vi "Message to Message Handler.vi"(0 "Message Handler In":refnum<class "Message Handler.lvclass">, 1 "CMD":T2, 2 "Type of Message":T1, 5 "Process":refnum<class "Process.lvclass">, 7 "Data In":variant, 9 "Return State":string, 11 "Error In":errorcluster, 12 "Timeout in ms (-1)":i32) -> (4 "Message Handler Out":refnum<class "Message Handler.lvclass">, 8 "Data Out":variant, 15 "Error Out":errorcluster)   [LabVIEW 2023, in "Message Handler.lvclass"]
uses:
  Message Handler.lvclass
  Public/Ctrls/CMDs.ctl
  Process/Process.lvclass
  Public/Ctrls/Type of Message.ctl
  Process/Process.lvclass/Process.ctl
  Message Handler.lvclass/Message Handler.ctl
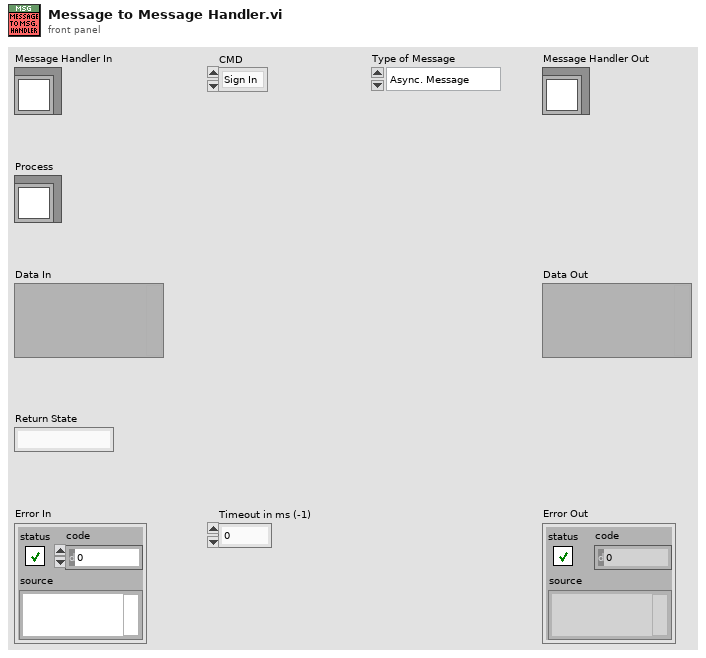
[diagram p1: front panel]
types:
  T1 = typedef "Message Handler.lvclass/Type of Message.ctl" = enum16{"Async. Message", "Async. Data Request", "Sync. Data Request"}
  T2 = typedef "Message Handler.lvclass/CMDs.ctl" = enum16{"Sign In"}
  T3 = typedef "ICanCommunicate.lvclass/Message.ctl" = cluster{"Sender Name":string, "Recipent Name":string, "Command":string, "Data":variant, "Time Stamp":timestamp, "GUID":string, "Chcecksum":string}
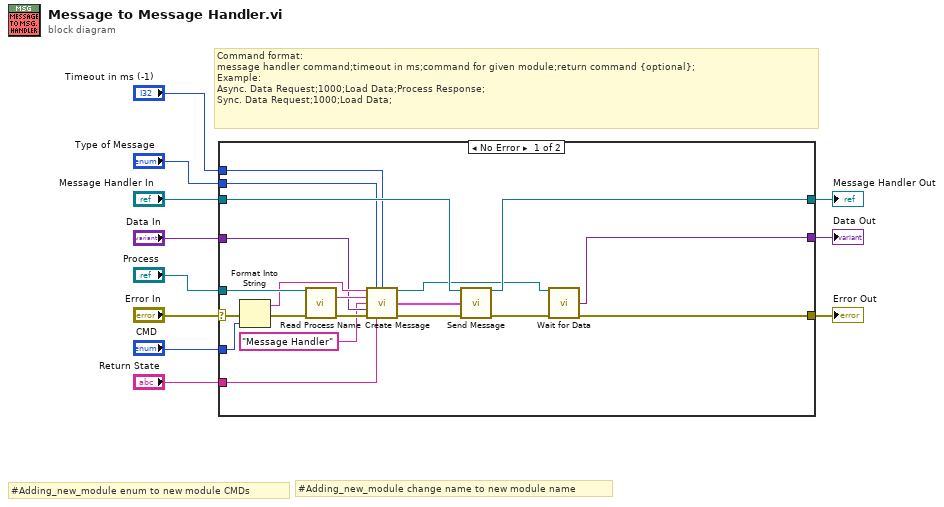
[diagram p0: block diagram]
diagram:
  # "Command format:\nmessage handler command;timeout in ms;command for given module;return command {optional};\nExample:\nAsync. Data Request;1000;Load Data;Process Response;\nSync. Data Request;1000;Load Data;"
  # "#Adding_new_module change name to new module name"
  # "#Adding_new_module enum to new module CMDs"
  n1 = case shown="No Error" "Error In" {
    selector: "Error In" -> [w22 w34]
    tunnel: [w15 w34] -> w10
    tunnel: "Data In" -> [w21 w32]
    tunnel: "CMD" -> [w31 _]
    tunnel: "Message Handler In" -> [w30 w33]
    tunnel: [w29 w33] -> w6
    tunnel: "Process" -> [w28 _]
    tunnel: "Timeout in ms (-1)" -> [w14 _]
    tunnel: "Type of Message" -> [w25 _]
    tunnel: "Return State" -> [w17 _]
    tunnel: [w12 w32] -> w1
    frame No Error {
      n2 = Format Into String(error in=w22, w31) -> (resulting string=w26:string, error out=w24:errorcluster)  [unwired: 2 in]
      n3 = call "Read Process Name.vi"("Process In"=w28, "Error In"=w24) -> ("Process Name"=w27:string, "Error Out"=w23:errorcluster)  [unwired: 11 in, 1 out]
      n4 = call "Create Message.vi"("CMD String"=w26, "Type of Message"=w25, "Timeout in ms (-1)"=w14, "Sender Name"=w27, "Recipent Name"="Message Handler" ("Recipent ID"), "Data"=w21, "Error In"=w23, "Return State"=w17) -> ("Wait Notifier"=w13:refnum<notifier>, "Message"=w19:T3, "Error Out"=w18:errorcluster)  [unwired: 5 in]
      n5 = call-dynamic "Send Message.vi"("ICanCommunicate In"=w30, "Message"=w19, "Error In"=w18) -> ("ICanCommunicate Out"=w29:refnum<class "Message Handler.lvclass">, "Error Out"=w16:errorcluster)  [unwired: 11 in]
      n6 = call "Wait for Data.vi"("Wait Notifier"=w13, "Error In"=w16) -> ("Data"=w12:variant, "Error Out"=w15:errorcluster)  [unwired: 12 in]
    }
    frame Error {
    }
  }
  "Error Out" <- w10
  "Message Handler Out" <- w6
  "Data Out" <- w1
